vi "UI.StationUpdate.vi"(8 "error in (no error)":errorcluster, 11 "state variables":T1) -> (0 "error out":errorcluster)   [LabVIEW 2015, in "Overview GUI.lvlib"]
uses:
  Overview GUI.lvlib
  Types/Overview.StateVariables.ctl
  <vilib>/NI Veristand/Execution/Workspace/WorkspaceAPI.ctl
  NationalInstruments.VeriStand.ClientAPI
  <vilib>/NI Veristand/Execution/Workspace/SystemStateRegEventRef.ctl
  <vilib>/NI Veristand/Execution/Workspace/Target State Info.ctl
  <vilib>/NI Veristand/Execution/Workspace/Target State.ctl
  <vilib>/NI Veristand/Execution/Workspace/SystemStateEventRef.ctl
  <vilib>/Utility/miscctls.llb/LVRowAndColumnTypeDef.ctl
  <vilib>/NI Veristand/Execution/Workspace/NI VeriStand - Get Multiple Channel Values.vi
  Shared/Shared.lvlib
  <vilib>/NI Veristand/Execution/Workspace/NI_VS Workspace ExecutionAPI.lvlib
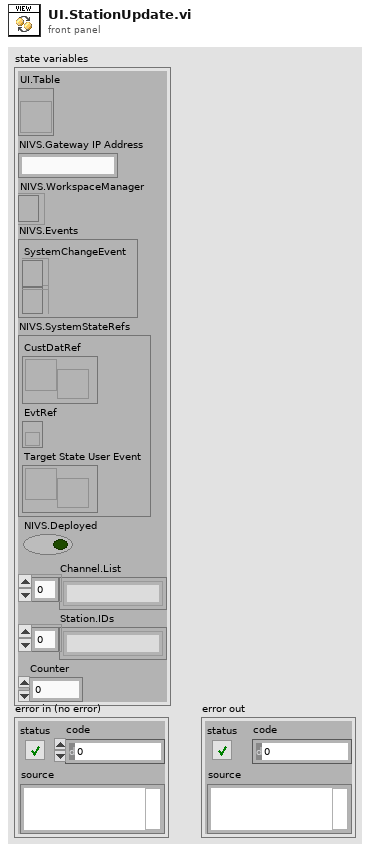
[diagram p1: front panel]
types:
  T1 = typedef "Overview GUI.lvlib/Overview.StateVariables.ctl" = cluster{"UI.Table":refnum<vi>, "NIVS.Gateway IP Address":string, "NIVS.WorkspaceManager":T2, "NIVS.Events":cluster{"SystemChangeEvent":T3, "WorkspaceEvent":refnum<event-registration>}, "NIVS.SystemStateRefs":T4, "NIVS.Deployed":bool, "Channel.List":string[], "Station.IDs":string[], "Counter":u8}
  T2 = typedef "NI_VS Workspace ExecutionAPI.lvlib/WorkspaceAPI.ctl" = refnum<k24>
  T3 = typedef "NI_VS Workspace ExecutionAPI.lvlib/SystemStateRegEventRef.ctl" = refnum<event-registration>
  T4 = typedef "NI_VS Workspace ExecutionAPI.lvlib/SystemStateEventRef.ctl" = cluster{"CustDatRef":refnum<user-event>, "EvtRef":refnum<k27>, "Target State User Event":refnum<user-event>}
  T5 = typedef "LVRowAndColumnTypeDef.ctl" = cluster{"Row":i32, "Column":i32}
  T6 = typedef "Single Station Execution.lvlib/Stimulus.Status.ctl" = cluster{"Restart":bool, "NIVS.SequenceState":T7, "Alarmed?":bool, "Disable?":bool}
  T7 = typedef "Single Station Execution.lvlib/Execution.SequenceState.ctl" = enum16{"Idle", "Initializing", "Running", "Paused", "Finalizing", "Complete"}
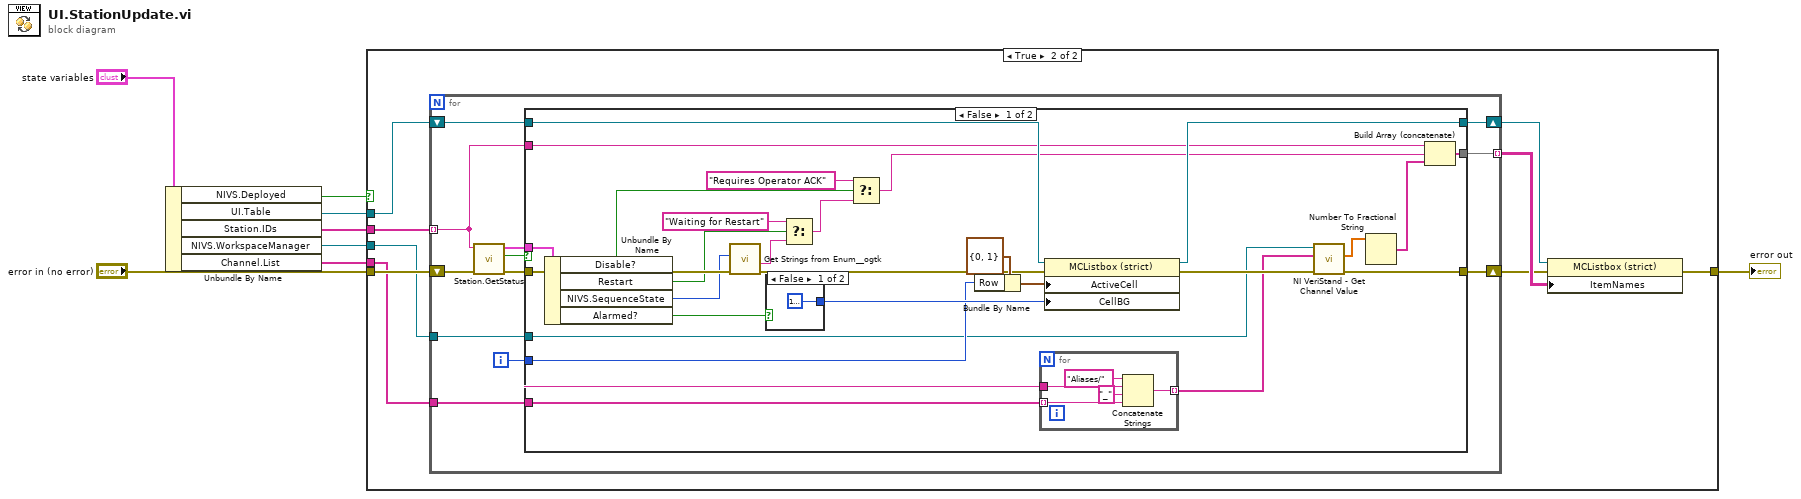
[diagram p0: block diagram]
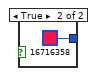
[diagram p3: hidden frame]
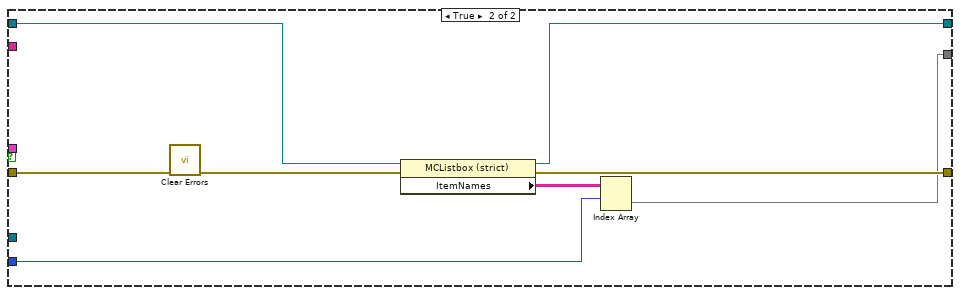
[diagram p4: hidden frame]
diagram:
  n1 = Unbundle By Name("state variables") -> ("NIVS.Deployed"=w1:bool, "UI.Table"=w7:refnum<vi>, "Station.IDs"=w8:string[], "NIVS.WorkspaceManager"=w4:T2, "Channel.List"=w3:string[])
  n2 = case shown="True" w1 {
    tunnel: w8 -> [_ w18]
    tunnel: w7 -> [_ w17]
    tunnel: "error in (no error)" -> [w9 w16]
    tunnel: w4 -> [_ w15]
    tunnel: w3 -> [_ w14]
    tunnel: [w9 w10] -> w2
    frame False {
    }
    frame True {
      n3 = for {
        shift-right: [w24] -> w11
        shift-left: w16 -> [w30]
        tunnel: w18 -> [w21] mode=indexing
        tunnel: [w25] -> w13 mode=indexing
        tunnel: w15 -> [w23]
        tunnel: w14 -> [w20]
        shift-right: [w22] -> w12
        shift-left: w17 -> [w29]
        i -> [w27]
        n4 = call "Station.GetStatus.vi"("error in (no error)"=w30, "Station.ID"=w21) -> ("error out"=w26:errorcluster, "timed out?"=w19:bool, "Station.Status"=w28:T6)  [unwired: 7 in]
        n5 = case shown="False" w19 {
          tunnel: w29 -> [w57 w71]
          tunnel: w28 -> [w56 _]
          tunnel: w27 -> [w53 w66]
          tunnel: w26 -> [w50 w72]
          tunnel: [w44 w65] -> w25
          tunnel: [w42 w69] -> w24
          tunnel: w23 -> [w41 _]
          tunnel: [w38 w68] -> w22
          tunnel: w21 -> [w37 _]
          tunnel: w20 -> [w36 _]
          frame False {
            n6 = Unbundle By Name(w56) -> ("Disable?"=w33:bool, "Restart"=w47:bool, "NIVS.SequenceState"=w48:T7, "Alarmed?"=w55:bool)
            n7 = call <userlib>:"Get Strings from Enum__ogtk.vi"("error in (no error)"=w50, "Enum"=w48) -> ("error out"=w49:errorcluster, "String Value"=w45:string)  [unwired: 6 in, 2 out]
            n8 = case shown="False" w55 {
              tunnel: [u32 16777216 u32 16716358] -> w54
              frame False {
              }
              frame True {
              }
            }
            n9 = Select(t="Waiting for Restart", s=w47, f=w45) -> (s? t:f=w32:string)
            n10 = Select(t="Requires Operator ACK", s=w33, f=w32) -> (s? t:f=w31:string)
            n11 = Bundle By Name(cluster=T5 {"Row"=0, "Column"=1} ("Active Cell:Active Cell"), "Row"=w53) -> (w51:T5)
            n12 = for {
              tunnel: w36 -> [w62] mode=indexing
              tunnel: w37 -> [w60]
              tunnel: [w58] -> w35 mode=indexing
              n13 = Concatenate Strings("Aliases/" ("string"), w60, "_" ("string"), w62) -> (w58:string)
            }
            n14 = property class="MCListbox (strict)"(reference=w57, error in=w49, "ActiveCell"=w51, "CellBG"=w54) -> (reference out=w38:refnum<vi>, error out=w43:errorcluster)
            n15 = call-poly <vilib>:"NI VeriStand - Get Channel Value.vi"("error in (no error)"=w43, "Channels"=w35, "WorkspaceManager in"=w41) -> ("error out"=w42:errorcluster, "Values"=w40:dbl[])  [unwired: 6 in, 1 out]
            n16 = Number To Fractional String(number=w40) -> (F-format string=w39:string[])  [unwired: 3 in]
            n17 = Build Array (concatenate)(w37, w31, w39) -> (w44:string[])
          }
          frame True {
            n18 = call <vilib>:"Clear Errors.vi"("error in (no error)"=w72) -> ("error out"=w70:errorcluster)  [unwired: 5 in, 1 out]
            n19 = property class="MCListbox (strict)"(reference=w71, error in=w70) -> (reference out=w68:refnum<vi>, error out=w69:errorcluster, "ItemNames"=w67:string[][])
            n20 = Index Array(array=w67, index (row)=w66) -> (element=w65:string[])  [unwired: 1 in]
          }
        }
      }
      n21 = property class="MCListbox (strict)"(reference=w12, error in=w11, "ItemNames"=w13) -> (error out=w10:errorcluster)  [unwired: 1 out]
    }
  }
  "error out" <- w2
